vi "ProgG_005_MG.vi"(1 "x2":ext=19.4, 2 "x1":ext=14.1) -> (0 "Y":dbl)   [LabVIEW 2021]
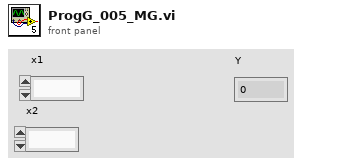
[diagram p1: front panel]
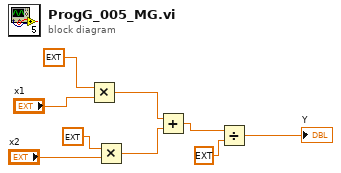
[diagram p0: block diagram]
diagram:
  n1 = Multiply(x=ext 0.9, y="x1") -> (x*y=w5:ext)
  n2 = Multiply(x=ext 0.8, y="x2") -> (x*y=w4:ext)
  n3 = Add(x=w5, y=w4) -> (x+y=w3:ext)
  n4 = Divide(x=w3, y=ext 2.0) -> (x/y=→"Y":ext)
